vi "insert into array.vi"() -> ()   [LabVIEW 2016]
panel:
  out "subarray":i32[](array[numeric])
  out "deleted portion 2":i32[][](array[numeric])
  out "array w/ subset deleted 2":i32[][][](array[numeric])
  out "appended array 2":i32[][][](array[numeric])
  in  "in array":i32[][][](array[numeric])
  out "appended array":i32[][](array[numeric])
  in  "Array 3":i32[](array[numeric])
  in  "index (row)":i32
  out "deleted portion":dbl[](array[numeric])
  out "array w/ subset deleted":dbl[][](array[numeric])
  out "Array 2":i32[](array[numeric])
  out "Numeric 3":i32
  out "Numeric 2":i32
  out "output array 2":dbl[](array[numeric])
  in  "Numeric":i32
  out "Array":i32[](array[numeric])
  out "output array":dbl[][](array[numeric])
  in  "new element/subarray":dbl[](array[numeric])
  in  "array":dbl[][](array[numeric])
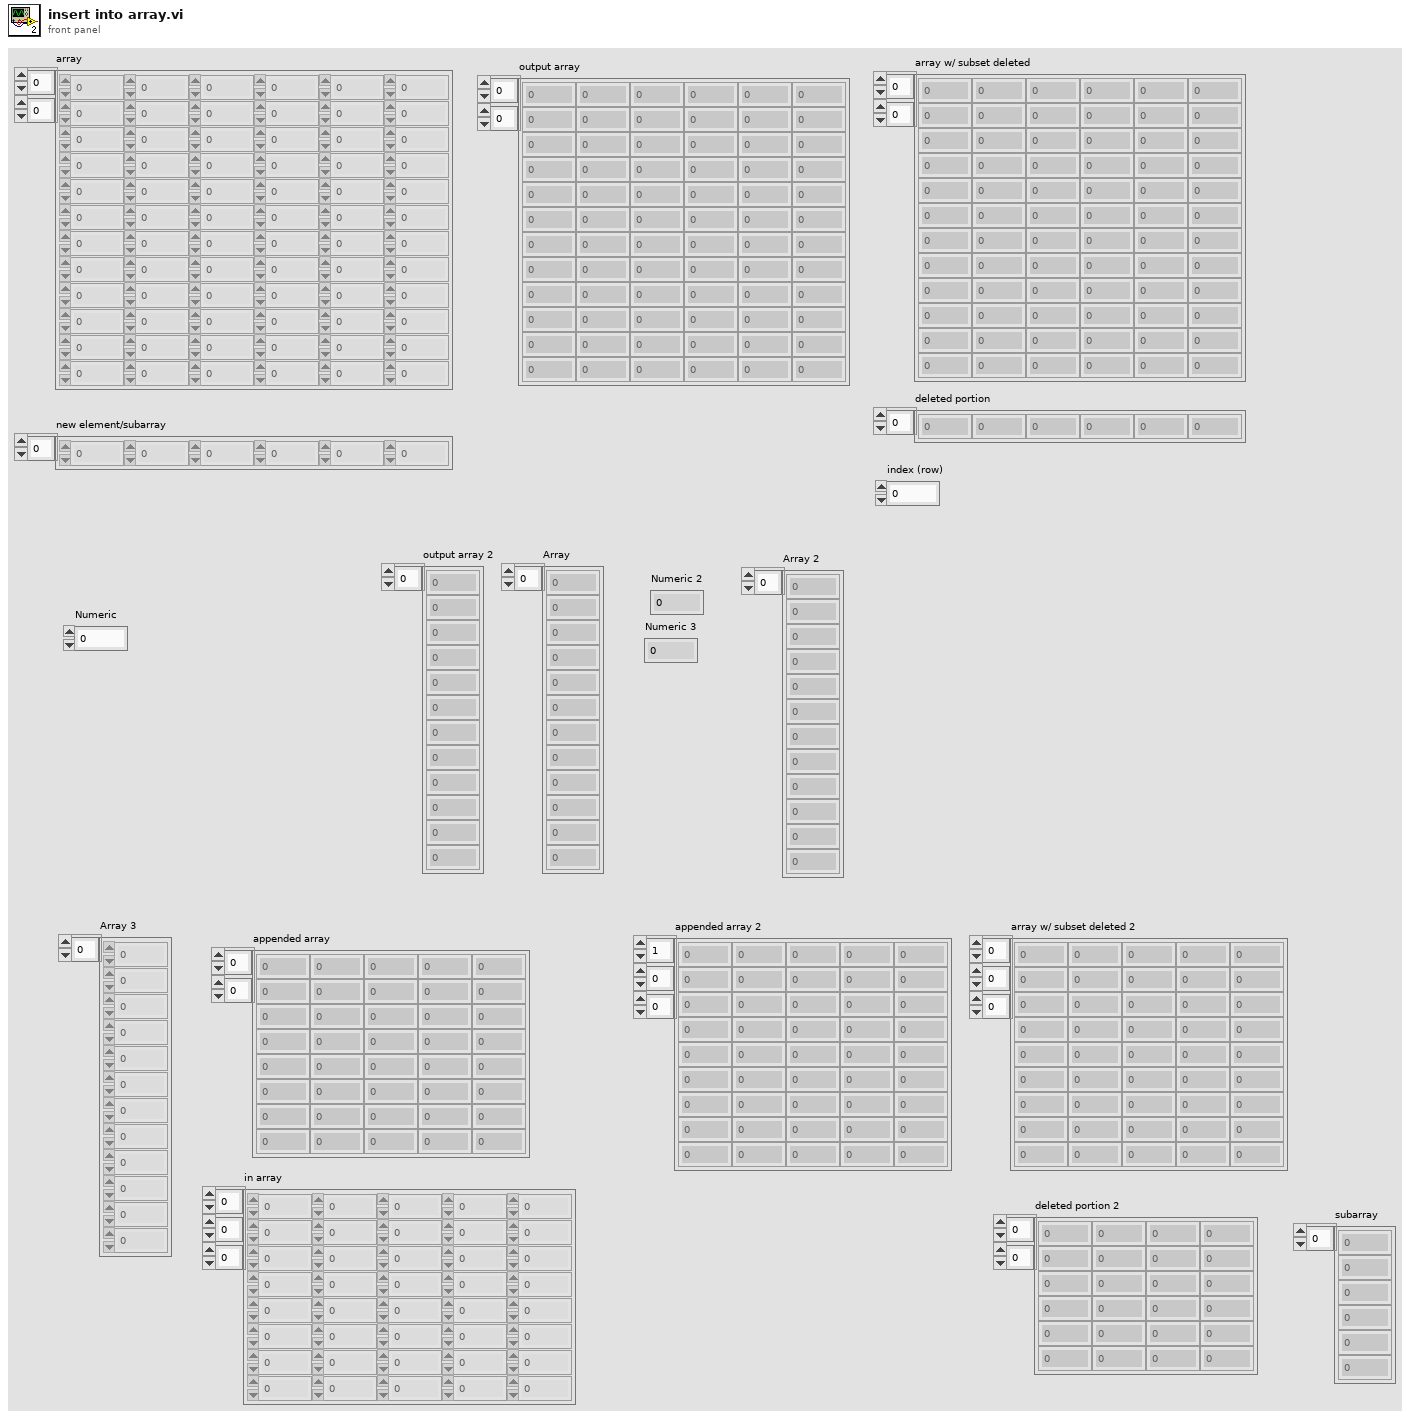
[diagram p1: front panel]
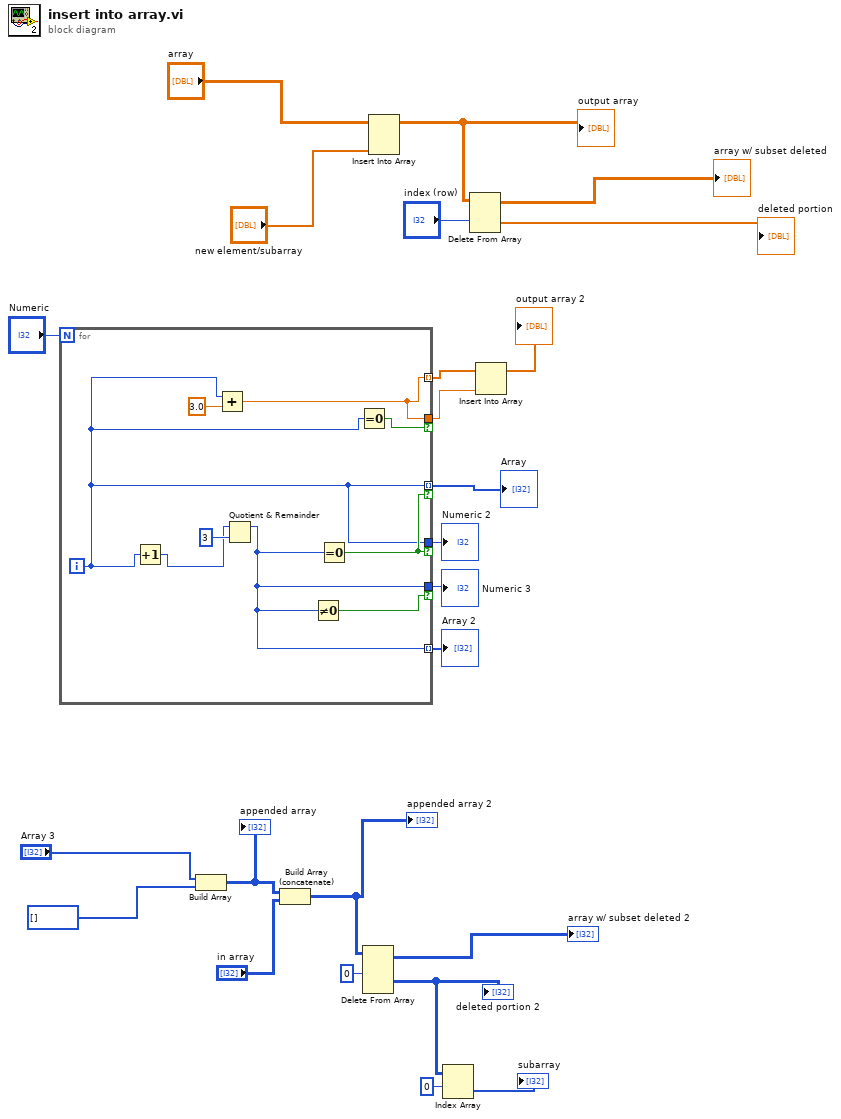
[diagram p0: block diagram]
diagram:
  n1 = for {
    N: "Numeric" -> [_]
    tunnel: [w26] -> w22 mode=indexing if=w29
    tunnel: [w30] -> w20 mode=indexing
    tunnel: [w30] -> w19 if=w32
    tunnel: [w26] -> w17 if=w29
    tunnel: [w27] -> w16 if=w28
    tunnel: [w27] -> w15 mode=indexing
    i -> [w26]
    n2 = Increment(x=w26) -> (x+1=w25:i32)
    n3 = Add(x=w26, y=3.0) -> (x+y=w30:dbl)
    n4 = Quotient & Remainder(x=w25, y=3) -> (x-y*floor(x/y)=w27:i32)  [unwired: 1 out]
    n5 = Not Equal To 0?(x=w27) -> (x != 0?=w28:bool)
    n6 = Equal To 0?(x=w27) -> (x = 0?=w29:bool)
    n7 = Equal To 0?(x=w26) -> (x = 0?=w32:bool)
  }
  "Array" <- w22
  "Numeric 2" <- w17
  "Numeric 3" <- w16
  "Array 2" <- w15
  n8 = Build Array("Array 3", i32[] [] ("element")) -> (w10:i32[][])
  "appended array" <- w10
  n9 = Build Array (concatenate)(w10, "in array") -> (w7:i32[][][])
  "appended array 2" <- w7
  n10 = Delete From Array "Delete From Array"(array=w7, index (dim 0)=0 ("index (page)")) -> (deleted portion=w3:i32[][], array with subset deleted=→"array w/ subset deleted 2":i32[][][])  [unwired: 3 in]
  "deleted portion 2" <- w3
  n11 = Insert Into Array "Insert Into Array"(array="array", new element="new element/subarray") -> (w14:dbl[][])  [unwired: 2 in]
  "output array" <- w14
  n12 = Index Array "Index Array"(array=w3, index (row)=0) -> (element=→"subarray":i32[])  [unwired: 1 in]
  n13 = Delete From Array(array=w14, index (row)="index (row)") -> (deleted portion=→"deleted portion":dbl[], array with subset deleted=→"array w/ subset deleted":dbl[][])  [unwired: 2 in]
  n14 = Insert Into Array "Insert Into Array"(array=w20, new element=w19) -> (→"output array 2":dbl[])  [unwired: 1 in]
